vi "Get String from User.vi"(8 "error in":errorcluster, 9 "timeout (s)":dbl=300.0, 10 "default value":string, 11 "prompt":string) -> (0 "error out":errorcluster, 1 "timeout?":bool, 2 "cancelled?":bool, 3 "string out":string)   [LabVIEW 2010]
panel:
  out "prompt display":string
  in  "user input":string
  in  "cancel btn":bool
  in  "OK btn":bool
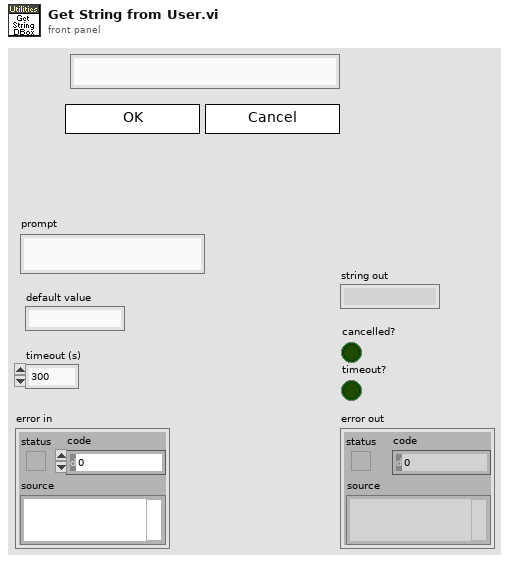
[diagram p1: front panel]
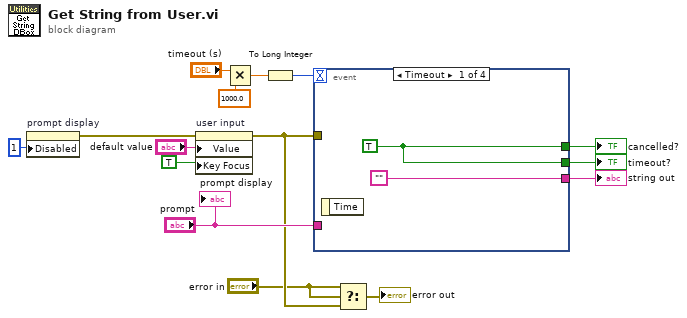
[diagram p0: block diagram]
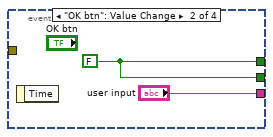
[diagram p2: hidden frame]
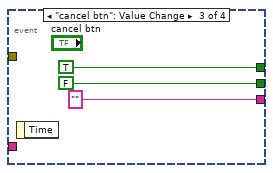
[diagram p3: hidden frame]
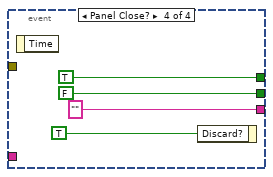
[diagram p4: hidden frame]
diagram:
  n1 = property on="prompt display" class="Str"("Disabled"=u8 1) -> (error out=w2:errorcluster)  [unwired: 2 in, 1 out]
  n2 = property on="user input" class="Str"(error in=w2, "Value"="default value", "Key Focus"=TRUE) -> (error out=w5:errorcluster)  [unwired: 1 in, 1 out]
  n3 = Multiply(x="timeout (s)", y=1000.0) -> (x*y=w12:dbl)
  n4 = To Long Integer(number=w12) -> (32bit integer=w13:i32)
  n5 = event shown="[0] Timeout" {
    selector: _ -> [_ _ _ _]
    dyn-events: _ -> [_ _ _ _]
    timeout: w13 -> [_ _ _ _]
    tunnel: w5 -> [_ _ _ _]
    tunnel: "prompt" -> [_ _ _ _]
    tunnel: [w17 w19 TRUE TRUE] -> w8
    tunnel: [w17 w19 FALSE FALSE] -> w7
    tunnel: ["" ("user input") "user input" "" ("user input") "" ("user input")] -> w6
    event Timeout {
      w17 = TRUE
      n6 = event-data() -> ()  [unwired: 2 out]
    }
    event "OK btn": Value Change {
      w19 = FALSE
      n7 = event-data() -> ()  [unwired: 2 out]
    }
    event "cancel btn": Value Change {
      n8 = event-data() -> ()  [unwired: 2 out]
    }
    event Panel Close? {
      n9 = event-data() -> ()  [unwired: 2 out]
      n10 = event-data("Discard?"=TRUE) -> ()  [unwired: 1 in, 1 out]
    }
  }
  "string out" <- w6
  "cancelled?" <- w8
  "timeout?" <- w7
  n11 = Select(t="error in", s="error in", f=w5) -> (s? t:f=→"error out":errorcluster)
  "prompt display" <- "prompt"
